vi "sm_MFLI_7004.vi"(8 "error in":errorcluster caption="entrée d'erreur", 9 "variant (data or path)":variant, 10 "address":string, 11 "cmd SM":T1) -> (0 "error out":errorcluster, 2 "Selected Device":string, 3 "return value":variant)   [LabVIEW 2018]
uses:
  Program Files/National Instruments/LabVIEW 2023/instr.lib/Zurich Instruments LabOne/Zurich Instruments LabOne.lvlib
  Program Files/National Instruments/LabVIEW 2023/instr.lib/Zurich Instruments LabOne/Public/Configure/ziGetValueDouble.vi
  Program Files/National Instruments/LabVIEW 2023/instr.lib/Zurich Instruments LabOne/Public/Configure/ziSetValueDouble.vi
  Program Files/National Instruments/LabVIEW 2023/instr.lib/Zurich Instruments LabOne/Public/Configure/ziGetValueDemodSampleEx.vi
  cmd_MFLI.ctl
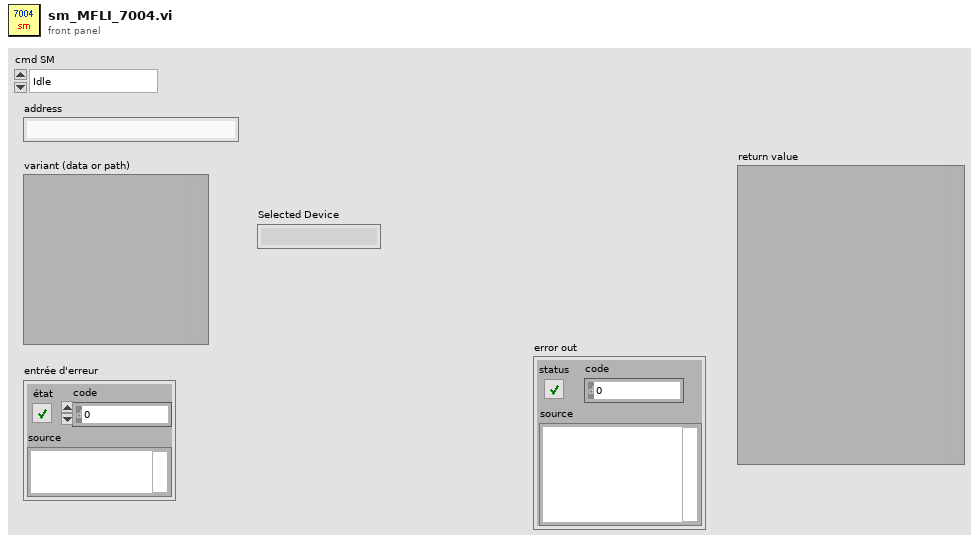
[diagram p1: front panel]
types:
  T1 = typedef "cmd_MFLI.ctl" = enum16{"Idle", "Open", "Read Config", "Save Config", "read_XY_demod_0", "spot_XY_demod_0", "read_XY_both", "spot_XY_both", "get_time_constant", "get_time_constants", "harmonic_1", "harmonic_3", "A", "A-B", "set_TC", "set_TCs", "sweep_2demods", "sweep_demod_0", "Locked ?", "Send Command", "autorange", "Error", "Close", "Exit"}
  T2 = typedef "Zurich Instruments LabOne.lvlib/ziTypeHandle.ctl" = cluster{"handleValid":bool, "Conn":u64, "Path Prefix":string, "Handle":u64, "Connected":bool, "Clockbase(s)":dbl}
  T3 = typedef "Zurich Instruments LabOne.lvlib/ziTypeDemodSampleSingle.ctl" = cluster{"Timestamps (ticks)":u64, "X (Vrms)":dbl, "Y (Vrms)":dbl, "Osc Phase (deg)":dbl, "Freq (Hz)":dbl, "DIO":u32, "AuxIn0 (V)":dbl, "AuxIn1 (V)":dbl, "Trigger":u32}
  T4 = typedef "Zurich Instruments LabOne.lvlib/ziTypeDemodSampleEx.ctl" = cluster{"Timestamps (ticks)":u64[], "X (Vrms)":dbl[], "Y (Vrms)":dbl[], "Osc Phase (rad)":dbl[], "Freq (Hz)":dbl[], "DIO":u32[], "Aux In 0 (V)":dbl[], "Aux In 1 (V)":dbl[], "Trigger":u32[]}
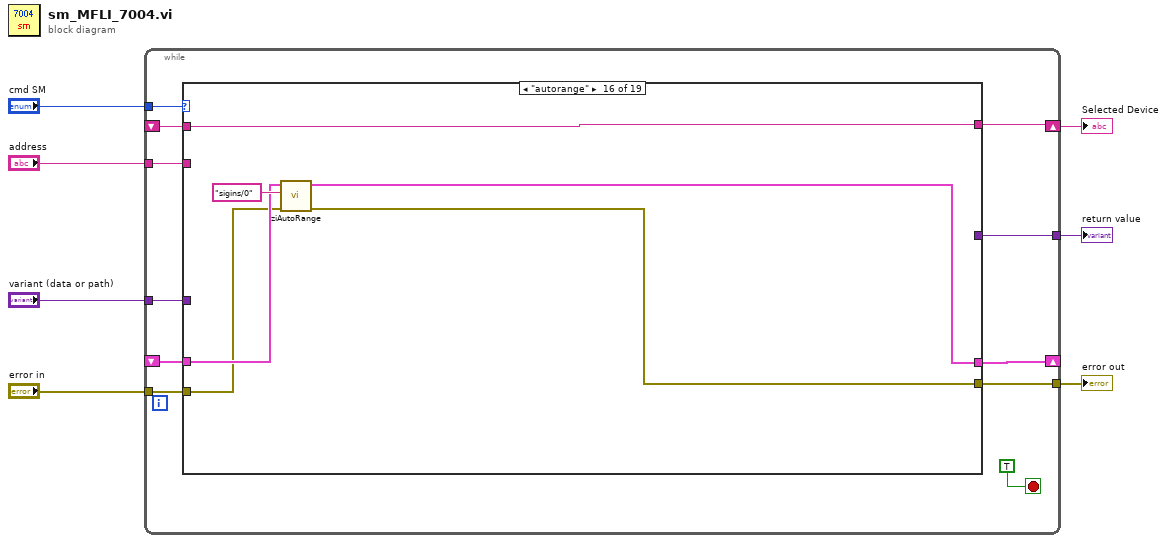
[diagram p0: block diagram]
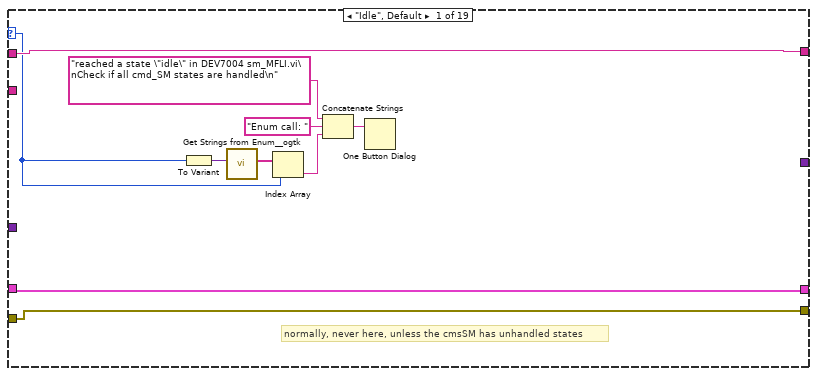
[diagram p2: hidden frame]
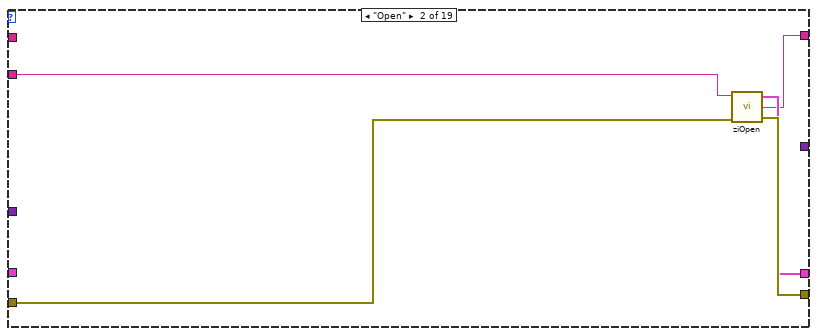
[diagram p3: hidden frame]
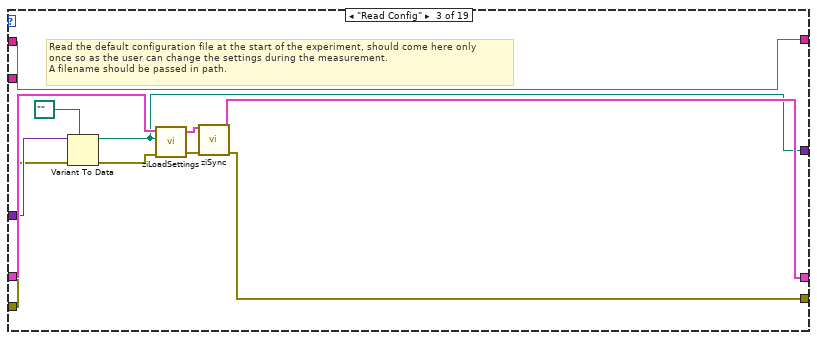
[diagram p4: hidden frame]
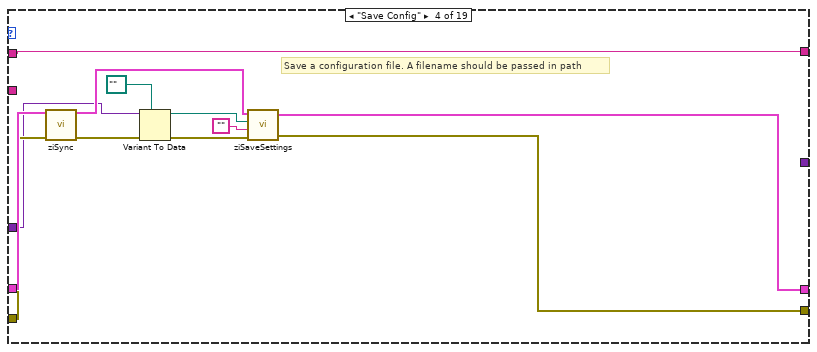
[diagram p5: hidden frame]
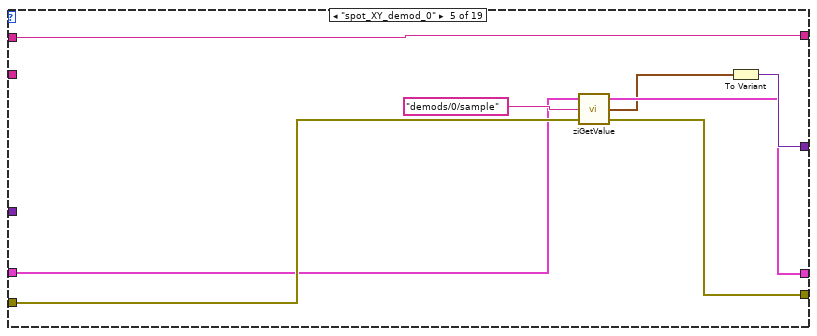
[diagram p6: hidden frame]
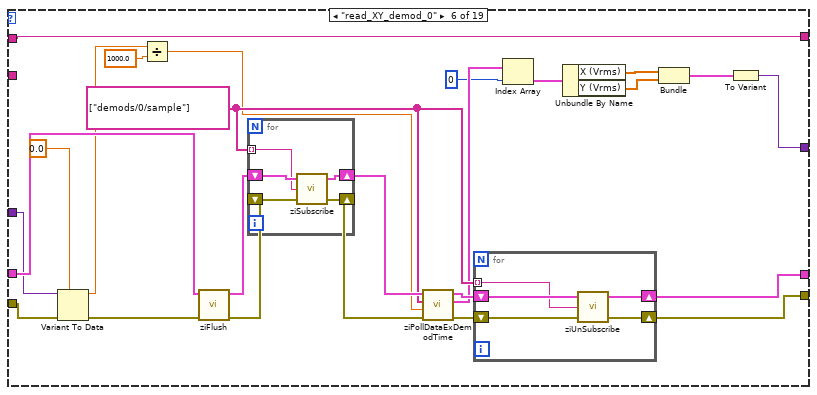
[diagram p7: hidden frame]
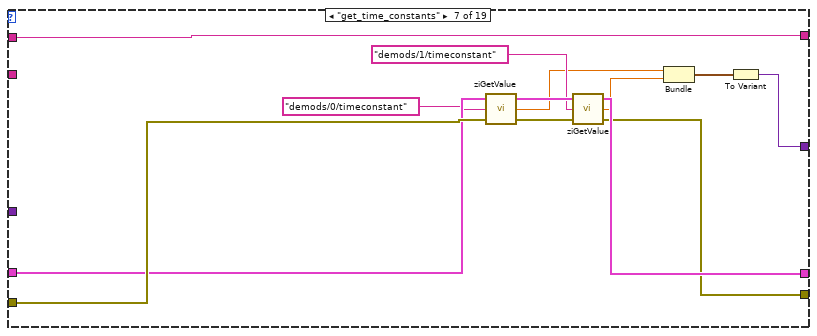
[diagram p8: hidden frame]
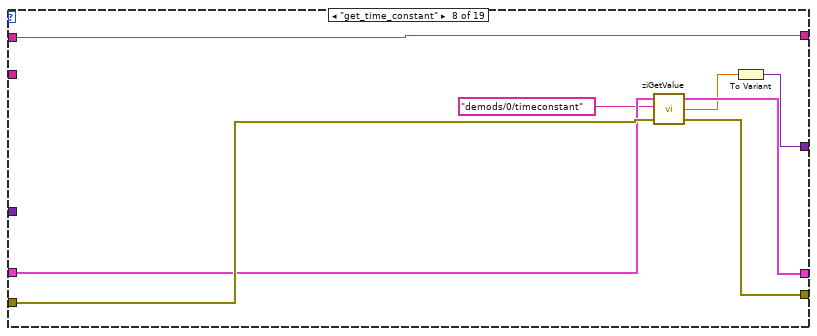
[diagram p9: hidden frame]
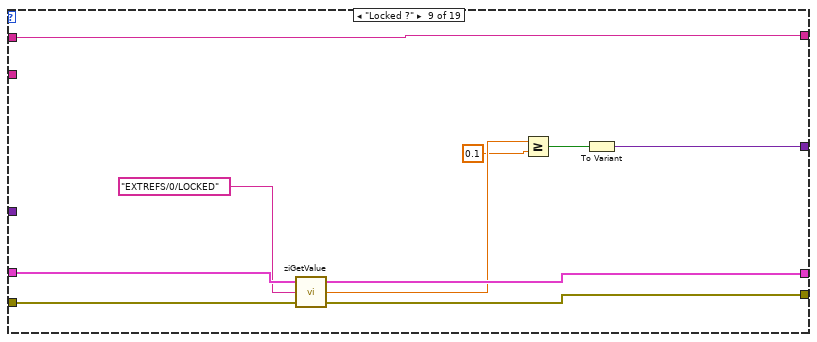
[diagram p10: hidden frame]
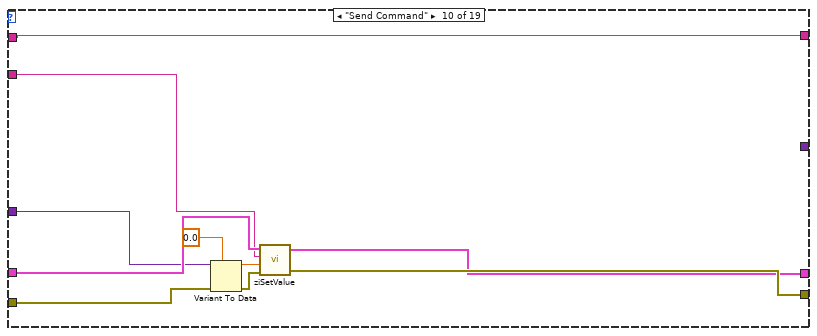
[diagram p11: hidden frame]
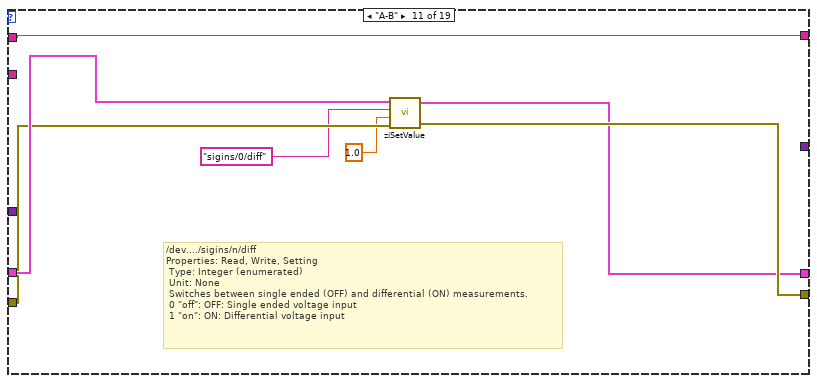
[diagram p12: hidden frame]
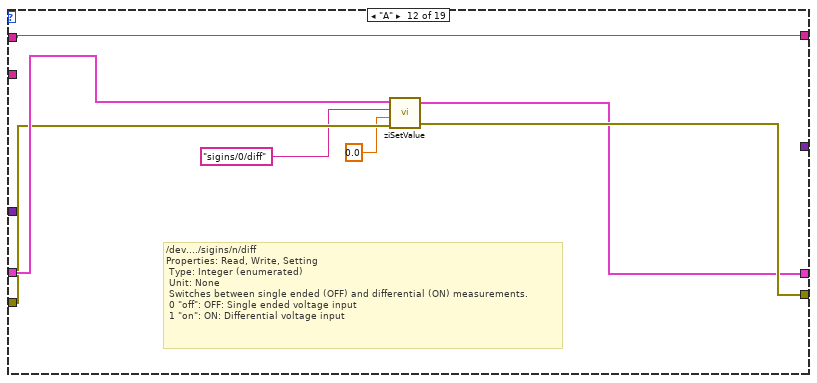
[diagram p13: hidden frame]
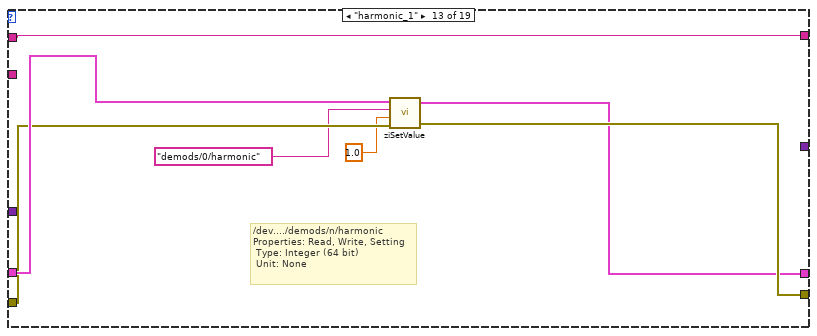
[diagram p14: hidden frame]
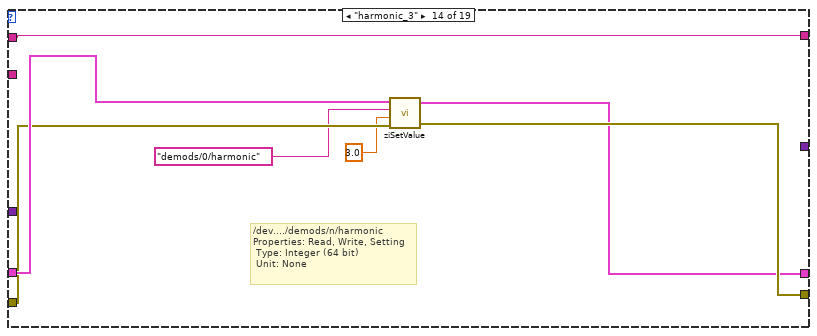
[diagram p15: hidden frame]
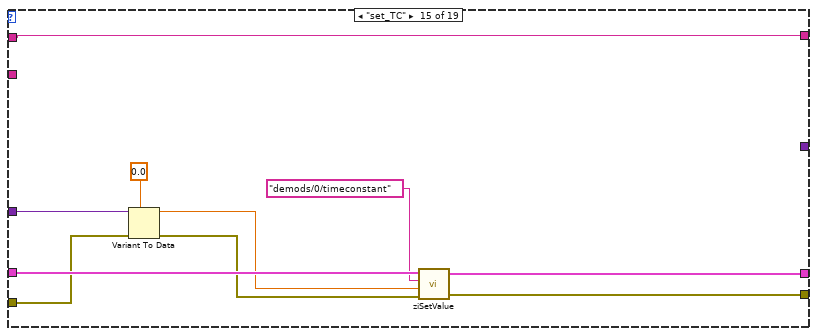
[diagram p16: hidden frame]
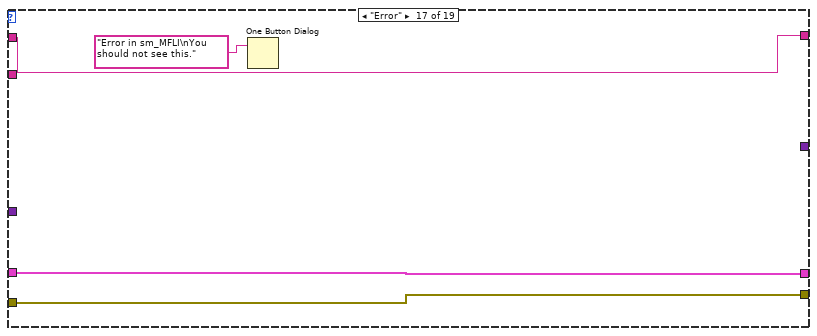
[diagram p17: hidden frame]
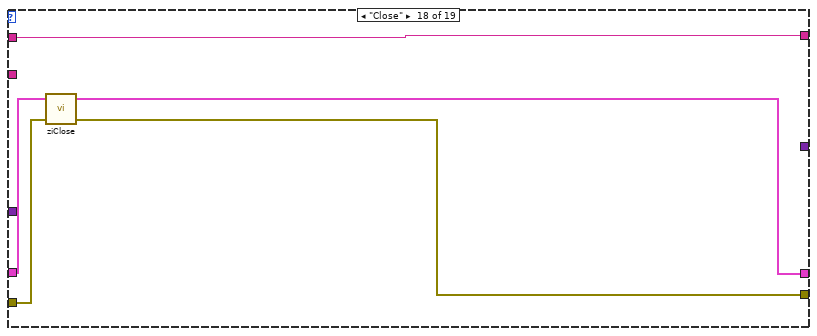
[diagram p18: hidden frame]
diagram:
  n1 = while {
    tunnel: "cmd SM" -> [w17]
    tunnel: "variant (data or path)" -> [w16]
    shift-right: [w13] -> _
    shift-left: _ -> [w12]
    tunnel: "address" -> [w11]
    tunnel: [w10] -> w3
    shift-right: [w9] -> w2
    shift-left: _ -> [w8]
    tunnel: "error in" -> [w14]
    tunnel: [w15] -> w1
    stop <- TRUE stop-if-true
    n2 = case shown="\"autorange\"" w17 {
      selector: w17 -> [w20 _ _ _ _ _ _ _ _ _ _ _ _ _ _ _ _ _ _]
      tunnel: w16 -> [_ _ w38 w48 _ w70 _ _ _ w137 _ _ _ _ w176 _ _ _ _]
      tunnel: [w23 w33 w42 w55 w58 w76 w104 w114 w129 w140 w147 w154 w161 w168 w178 w181 w188 w190 w195] -> w15
      tunnel: w14 -> [w23 w31 w35 w51 w62 w71 w112 w120 w130 w133 w145 w152 w159 w166 w172 w179 w188 w193 w195]
      tunnel: [w28 w32 w43 w54 w59 w75 w106 w115 w126 w132 w144 w151 w158 w165 w171 w182 w186 w191 w196] -> w13
      tunnel: w12 -> [w28 _ w44 w52 w60 w77 w111 w119 w128 w139 w146 w153 w160 w167 w177 w180 w186 w192 w196]
      tunnel: w11 -> [_ w29 _ _ _ _ _ _ _ w138 _ _ _ _ _ _ _ _ _]
      tunnel: [_ _ w34 _ w64 w89 w109 w117 w123 _ _ _ _ _ _ _ _ _ _] -> w10
      tunnel: [w27 w30 w40 w50 w63 w88 w108 w116 w121 w131 w143 w150 w157 w164 w170 w184 w185 w189 w194] -> w9
      tunnel: w8 -> [w27 _ w40 w50 w63 w88 w108 w116 w121 w131 w143 w150 w157 w164 w170 w184 w185 w189 w194]
      frame "Idle", Default {
        # "normally, never here, unless the cmsSM has unhandled states"
        n3 = To Variant(anything=w20) -> (Variant=w22:variant)
        n4 = call "Get Strings from Enum__ogtk.vi"("Enum"=w22) -> ("Enum Strings"=w21:string[])  [unwired: 7 in, 3 out]
        n5 = Index Array(array=w21, index=w20) -> (element=w19:string)
        n6 = Concatenate Strings("reached a state \"idle\" in DEV7004 sm_MFLI.vi\nCheck if all cmd_SM states are handled\n" ("message"), "Enum call: ", w19) -> (w25:string)
        n7 = One Button Dialog(message=w25) -> ()  [unwired: 1 in, 1 out]
      }
      frame "Open" {
        n8 = call "ziOpen.vi"("Error In"=w31, "Address"=w29) -> ("Error Out"=w33:errorcluster, "Selected Device"=w30:string, "HandleOut"=w32:T2)  [unwired: 2 in]
      }
      frame "Read Config" {
        # "Read the default configuration file at the start of the experiment, should come here only\nonce so as the user can change the settings during the measurement. \nA filename should be passed in path."
        n9 = Variant To Data(error in=w35, type=path "" ("Application Directory"), Variant=w38) -> (data=w34:path, error out=w36:errorcluster)
        n10 = call "ziLoadSettings.vi"("Error in"=w36, "File path (dialog if empty)"=w34, "Handle in"=w44) -> ("Error out"=w39:errorcluster, "Handle out"=w41:T2)  [unwired: 2 in]
        n11 = call "ziSync.vi"("Handle In"=w41, "Error In"=w39) -> ("Handle Out"=w43:T2, "Error Out"=w42:errorcluster)  [unwired: 12 in]
      }
      frame "Save Config" {
        # "Save a configuration file. A filename should be passed in path"
        n12 = call "ziSync.vi"("Handle In"=w52, "Error In"=w51) -> ("Handle Out"=w53:T2, "Error Out"=w46:errorcluster)  [unwired: 12 in]
        n13 = Variant To Data(error in=w46, type=path "" ("Application Directory"), Variant=w48) -> (data=w47:path, error out=w45:errorcluster)
        n14 = call "ziSaveSettings.vi"("Error In"=w45, "Path (\"\")"="", "file path (dialog if empty)"=w47, "Handle In"=w53) -> ("Error Out"=w55:errorcluster, "Handle Out"=w54:T2)  [unwired: 1 out]
      }
      frame "spot_XY_demod_0" {
        n15 = call-poly "ziGetValue.vi"("error in"=w62, "Path"="demods/0/sample", "Handle In"=w60) -> ("error out"=w58:errorcluster, "Demod Sample Out"=w57:T3, "Handle Out"=w59:T2)
        n16 = To Variant(anything=w57) -> (Variant=w64:variant)
      }
      frame "read_XY_demod_0" {
        w83 = string[] ["demods/0/sample"]
        n17 = Variant To Data(error in=w71, type=0.0, Variant=w70) -> (data=w67:dbl, error out=w69:errorcluster)
        n18 = Divide(x=w67, y=1000.0) -> (x/y=w65:dbl)
        n19 = call "ziFlush.vi"("error in"=w69, "Handle In"=w77) -> ("error out"=w81:errorcluster, "Handle Out"=w82:T2)  [unwired: 8 in]
        n20 = for {
          shift-right: [w97] -> w87
          shift-left: w81 -> [w98]
          shift-right: [w95] -> w86
          shift-left: w82 -> [w99]
          tunnel: w83 -> [w96] mode=indexing
          n21 = call "ziSubscribe.vi"("error in"=w98, "Path ()"=w96, "Handle In"=w99) -> ("error out"=w97:errorcluster, "Handle Out"=w95:T2)  [unwired: 1 in]
        }
        n22 = call "ziPollDataExDemodTime.vi"("error in"=w87, "recording time (1) [s]"=w65, "SubscribepathArray"=w83, "Handle In"=w86) -> ("error out"=w85:errorcluster, "Demod Sample Out"=w80:T4[], "Handle Out"=w84:T2)  [unwired: 5 in]
        n23 = for {
          shift-right: [w93] -> w76
          shift-left: w85 -> [w92]
          shift-right: [w94] -> w75
          shift-left: w84 -> [w91]
          tunnel: w83 -> [w90] mode=indexing
          n24 = call "ziUnSubscribe.vi"("error in"=w92, "Path (\"/\")"=w90, "Handle in"=w91) -> ("error out"=w93:errorcluster, "Handle out"=w94:T2)  [unwired: 1 in]
        }
        n25 = Index Array(array=w80, index=0 ("indice")) -> (element=w78:T4)
        n26 = Unbundle By Name(w78) -> ("X (Vrms)"=w74:dbl[], "Y (Vrms)"=w73:dbl[])
        n27 = Bundle("X (Vrms)"=w74, "Y (Vrms)"=w73) -> (w72:cluster{"X (Vrms)":dbl[], "Y (Vrms)":dbl[]})  [unwired: 1 in]
        n28 = To Variant(anything=w72) -> (Variant=w89:variant)
      }
      frame "get_time_constants" {
        n29 = call-poly "ziGetValue.vi"("error in"=w112, "Path"="demods/0/timeconstant", "Handle in"=w111) -> ("error out"=w105:errorcluster, "Value"=w102:dbl, "Handle out"=w107:T2)
        n30 = call-poly "ziGetValue.vi"("error in"=w105, "Path"="demods/1/timeconstant", "Handle in"=w107) -> ("error out"=w104:errorcluster, "Value"=w101:dbl, "Handle out"=w106:T2)
        n31 = Bundle("Value"=w102, "Value"=w101) -> (w100:cluster{"Value":dbl, "Value":dbl})  [unwired: 1 in]
        n32 = To Variant(anything=w100) -> (Variant=w109:variant)
      }
      frame "get_time_constant" {
        n33 = call-poly "ziGetValue.vi"("error in"=w120, "Path"="demods/0/timeconstant", "Handle in"=w119) -> ("error out"=w114:errorcluster, "Value"=w113:dbl, "Handle out"=w115:T2)
        n34 = To Variant(anything=w113) -> (Variant=w117:variant)
      }
      frame "Locked ?" {
        n35 = call-poly "ziGetValue.vi"("error in"=w130, "Path"="EXTREFS/0/LOCKED", "Handle in"=w128) -> ("error out"=w129:errorcluster, "Value"=w125:dbl, "Handle out"=w126:T2)
        n36 = Greater Or Equal?(x=w125, y=0.1) -> (x >= y?=w122:bool)
        n37 = To Variant(anything=w122) -> (Variant=w123:variant)
      }
      frame "Send Command" {
        n38 = Variant To Data(error in=w133, type=0.0 ("Value"), Variant=w137) -> (data=w135:dbl, error out=w134:errorcluster)
        n39 = call-poly "ziSetValue.vi"("Error In"=w134, "Value"=w135, "Path"=w138, "Handle In"=w139) -> ("Error Out"=w140:errorcluster, "Handle Out"=w132:T2)  [unwired: 1 in]
      }
      frame "A-B" {
        # "/dev..../sigins/n/diff \nProperties: Read, Write, Setting\n Type: Integer (enumerated)\n Unit: None\n Switches between single ended (OFF) and differential (ON) measurements.\n 0 \"off\": OFF: Single ended voltage input\n 1 \"on\": ON: Differential voltage input"
        n40 = call-poly "ziSetValue.vi"("Error In"=w145, "Value"=1.0, "Path"="sigins/0/diff", "Handle In"=w146) -> ("Error Out"=w147:errorcluster, "Handle Out"=w144:T2)  [unwired: 1 in]
      }
      frame "A" {
        # "/dev..../sigins/n/diff \nProperties: Read, Write, Setting\n Type: Integer (enumerated)\n Unit: None\n Switches between single ended (OFF) and differential (ON) measurements.\n 0 \"off\": OFF: Single ended voltage input\n 1 \"on\": ON: Differential voltage input"
        n41 = call-poly "ziSetValue.vi"("Error In"=w152, "Value"=0.0, "Path"="sigins/0/diff", "Handle In"=w153) -> ("Error Out"=w154:errorcluster, "Handle Out"=w151:T2)  [unwired: 1 in]
      }
      frame "harmonic_1" {
        # "/dev..../demods/n/harmonic \nProperties: Read, Write, Setting\n Type: Integer (64 bit)\n Unit: None"
        n42 = call-poly "ziSetValue.vi"("Error In"=w159, "Value"=1.0, "Path"="demods/0/harmonic", "Handle In"=w160) -> ("Error Out"=w161:errorcluster, "Handle Out"=w158:T2)  [unwired: 1 in]
      }
      frame "harmonic_3" {
        # "/dev..../demods/n/harmonic \nProperties: Read, Write, Setting\n Type: Integer (64 bit)\n Unit: None"
        n43 = call-poly "ziSetValue.vi"("Error In"=w166, "Value"=3.0, "Path"="demods/0/harmonic", "Handle In"=w167) -> ("Error Out"=w168:errorcluster, "Handle Out"=w165:T2)  [unwired: 1 in]
      }
      frame "set_TC" {
        n44 = Variant To Data(error in=w172, type=0.0 ("Value"), Variant=w176) -> (data=w174:dbl, error out=w173:errorcluster)
        n45 = call-poly "ziSetValue.vi"("Error In"=w173, "Value"=w174, "Path"="demods/0/timeconstant", "Handle In"=w177) -> ("Error Out"=w178:errorcluster, "Handle Out"=w171:T2)  [unwired: 1 in]
      }
      frame "autorange" {
        n46 = call "ziAutoRange.vi"("Error in"=w179, "Path"="sigins/0", "Handle in"=w180) -> ("Error out"=w181:errorcluster, "Handle out"=w182:T2)  [unwired: 6 in, 1 out]
      }
      frame "Error" {
        n47 = One Button Dialog(message="Error in sm_MFLI\nYou should not see this.") -> ()  [unwired: 1 in, 1 out]
      }
      frame "Close" {
        n48 = call "ziClose.vi"("Error In"=w193, "Handle In"=w192) -> ("Error Out"=w190:errorcluster, "Handle Out"=w191:T2)  [unwired: 2 in]
      }
      frame "Exit" {
        # "flush and clean up stuff"
      }
    }
  }
  "return value" <- w3
  "Selected Device" <- w2
  "error out" <- w1
